vi "start.vi"(8 "error in (no error)":errorcluster, 11 "Analog_Output in":refnum<class "Analog_Output.lvclass">) -> (0 "error out":errorcluster, 3 "Analog_Output out":refnum<class "Analog_Output.lvclass">)   [LabVIEW 2013, in "Analog_Output.lvclass"]
uses:
  Analog_Output.lvclass
  Analog_Output.lvclass/Analog_Output.ctl
  Experiment/Globals.vi
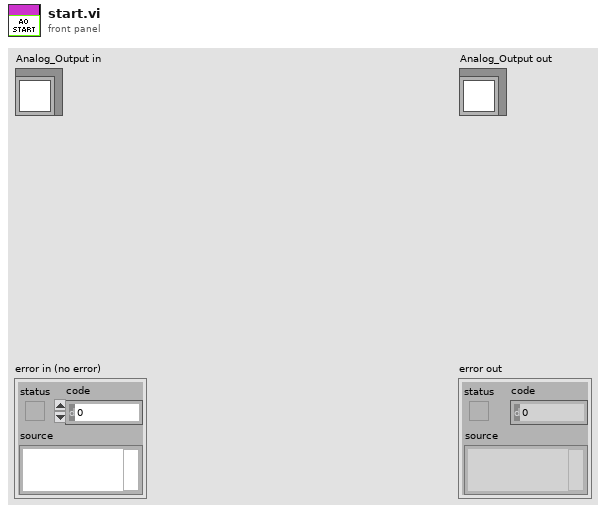
[diagram p1: front panel]
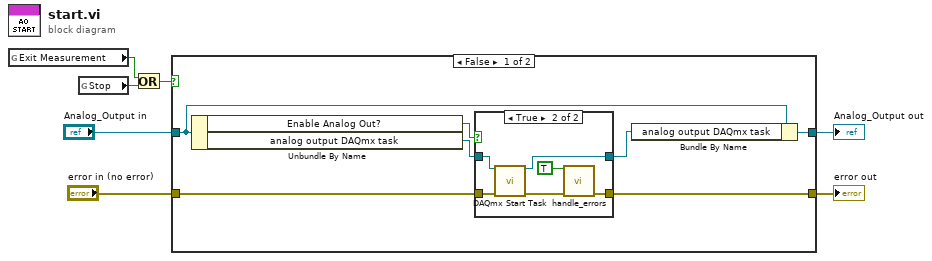
[diagram p0: block diagram]
diagram:
  n1 = global read "Globals.vi" "Exit Measurement"() -> (w3:bool)
  n2 = global read "Globals.vi" "Stop"() -> (w4:bool)
  n3 = Or(x=w3, y=w4) -> (x .or. y?=w2:bool)
  n4 = case shown="False" w2 {
    tunnel: [w8 w23] -> w7
    tunnel: [w10 w24] -> w5
    tunnel: "Analog_Output in" -> [w12 w24]
    tunnel: "error in (no error)" -> [w9 w23]
    frame False {
      n5 = Unbundle By Name(w12) -> ("Enable Analog Out?"=w14:bool, "analog output DAQmx task"=w13:refnum<k21>)
      n6 = case shown="True" w14 {
        tunnel: w13 -> [w16 w22]
        tunnel: [w16 w21] -> w11
        tunnel: [w15 w18] -> w8
        tunnel: w9 -> [w15 w20]
        frame False {
        }
        frame True {
          n7 = call <vilib>:"DAQmx Start Task.vi"("task/channels in"=w22, "error in"=w20) -> ("task out"=w21:refnum<k21>, "error out"=w17:errorcluster)  [unwired: 12 in]
          n8 = call "handle_errors.vi"("Exit Measurement"=TRUE, "error in (no error)"=w17) -> ("error out"=w18:errorcluster)  [unwired: 13 in]
        }
      }
      n9 = Bundle By Name(cluster=w12, "analog output DAQmx task"=w11) -> (w10:refnum<class "Analog_Output.lvclass">)
    }
    frame True {
    }
  }
  "error out" <- w7
  "Analog_Output out" <- w5
